vi "ROOT - Release Session.vi"(0 "OBJ - Session in":refnum<class "Session - Root.lvclass">, 5 "Session Handle in":T1, 11 "error in (no error)":errorcluster, 13 "force destroy? (F)":bool) -> (4 "OBJ - Session out":refnum<class "Session - Root.lvclass">, 15 "error out":errorcluster)   [LabVIEW 2015, in "Session - Root.lvclass"]
doc: "Initializes a measurement session\n\nSession data is set to the default values from \"set Defaults.vi\""
uses:
  Session - Root.lvclass
  Typedefs/Session Handle.ctl
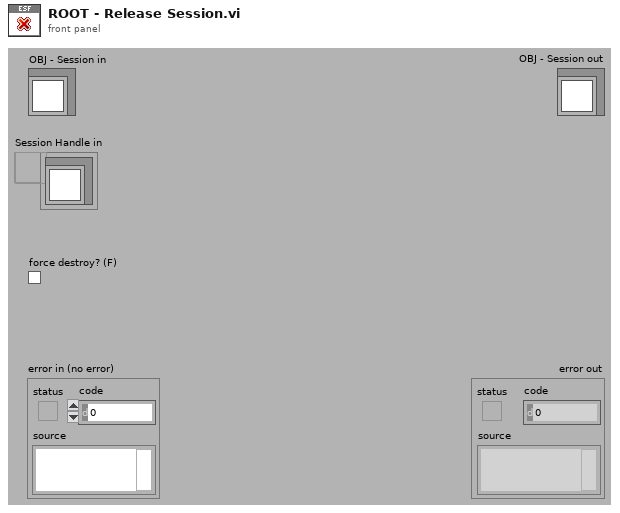
[diagram p1: front panel]
types:
  T1 = typedef "Session - Root.lvclass/Session Handle.ctl" = refnum<data-value>
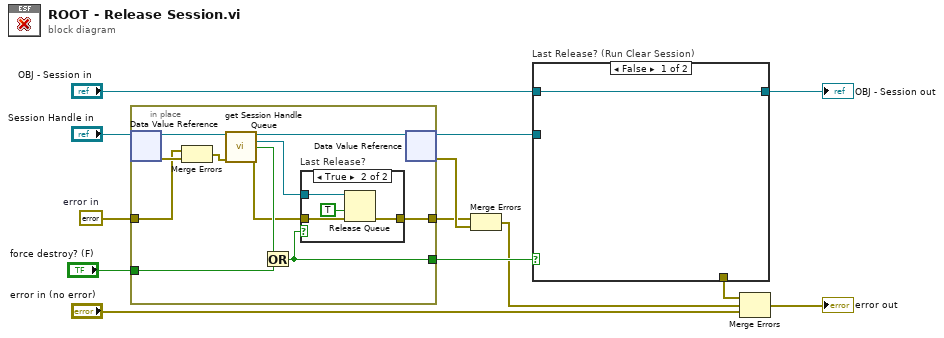
[diagram p0: block diagram]
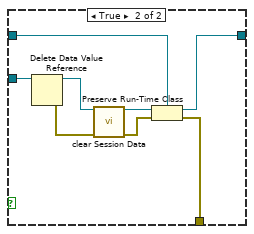
[diagram p3: hidden frame]
diagram:
  w6 = errorcluster {"status"=FALSE, "code"=0, "source"=""}  # error in
  n1 = in-place {
    in-place-border: [w14] -> w4
    in-place-border: "force destroy? (F)" -> [w16]
    in-place-border: w6 -> [w19]
    in-place-border: [w17] -> w5
    n2 = in-place-dvr #1("Session Handle in") -> (w24:refnum<class "Session - Root.lvclass">, w21:errorcluster)
    n3 = Merge Errors(w19, w21) -> (w20:errorcluster)
    n4 = call "get Session Handle Queue.vi"("OBJ - Session in"=w24, "error in (no error)"=w20) -> ("OBJ - Session out"=w23:refnum<class "Session - Root.lvclass">, "Session Queue Handle"=w18:refnum<queue>, "Last Session?"=w22:bool, "error out"=w15:errorcluster)  [unwired: 10 in]
    n5 = Or(x=w22, y=w16) -> (x .or. y?=w14:bool)
    n6 = case "Last Release?" shown="True" w14 {
      tunnel: w18 -> [_ w29]
      tunnel: [w25 w28] -> w17
      tunnel: w15 -> [w25 w27]
      frame False {
      }
      frame True {
        n7 = Release Queue(queue=w29, force destroy? (F)=TRUE, error in (no error)=w27) -> (error out=w28:errorcluster)  [unwired: 2 out]
      }
    }
    n8 = in-place-dvr #1(w23) -> (w9:T1, w8:errorcluster)
  }
  n9 = Merge Errors(w5, w8) -> (w1:errorcluster)
  n10 = case "Last Release? (Run Clear Session)" shown="False" w4 {
    tunnel: "OBJ - Session in" -> [w30 w36]
    tunnel: [w30 w33] -> w12
    tunnel: w9 -> [_ w38]
    tunnel: [_ w31] -> w3
    frame False {
    }
    frame True {
      n11 = Delete Data Value Reference(data value reference=w38) -> (data value=w37:refnum<class "Session - Root.lvclass">, error out=w32:errorcluster)  [unwired: 1 in]
      n12 = call-dynamic "clear Session Data.vi"("OBJ - Measurement Session in"=w37, "error in"=w32) -> ("OBJ - Measurement Session out"=w34:refnum<class "Session - Root.lvclass">, "error out"=w35:errorcluster)  [unwired: 12 in]
      n13 = Preserve Run-Time Class(object in=w34, error in=w35, 2:w36) -> (object out=w33:refnum<class "Session - Root.lvclass">, error out=w31:errorcluster)
    }
  }
  "OBJ - Session out" <- w12
  n14 = Merge Errors(w3, w1, "error in (no error)") -> (→"error out":errorcluster)
